vi "Parse Measured Data.vi"(6 "Waveform Template":waveform(dbl), 8 "error in":errorcluster, 9 "Current":dbl[](array[numeric]), 10 "Voltage":dbl[](array[numeric]), 11 "Electronic Load in":refnum<class "Electronic Load.lvclass">) -> (0 "error out":errorcluster, 3 "Electronic Load out":refnum<class "Electronic Load.lvclass">)   [LabVIEW 2019, in "Electronic Load.lvlib" / "Electronic Load.lvclass"]
uses:
  Library/Electronic Load.lvclass
  C:/Users/Public/Documents/Development/builds/Instruments/Instruments.lvlibp/Library/Instruments.lvclass
  Library/Electronic Load.lvclass/Electronic Load.ctl
  GUI/Read Measured_Table.vi
  GUI/Read Channel_Names.vi
  Accessors/Status/Read Status_Flags.vi
  GUI/Write Measured_Table.vi
  builds/Instruments/Instruments.lvlibp/Accessors/Write Measured.vi
  builds/Instruments/Instruments.lvlibp/Library/Instruments.lvclass
panel:
  in  "Waveform Labels":T1(ring)
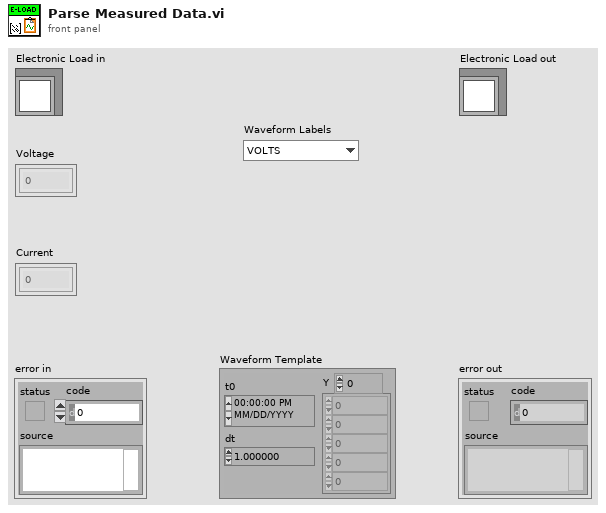
[diagram p1: front panel]
types:
  T1 = enum16{"VOLTS", "AMPS", "POWER", "OUTPUT", "OCP", "OVP"}
  T2 = typedef "Electronic Load.lvlib/Electronic Load.lvclass/Status_Flags.ctl" = cluster{"Interlock":bool, "OVP":bool, "OCP":bool, "Output":bool}
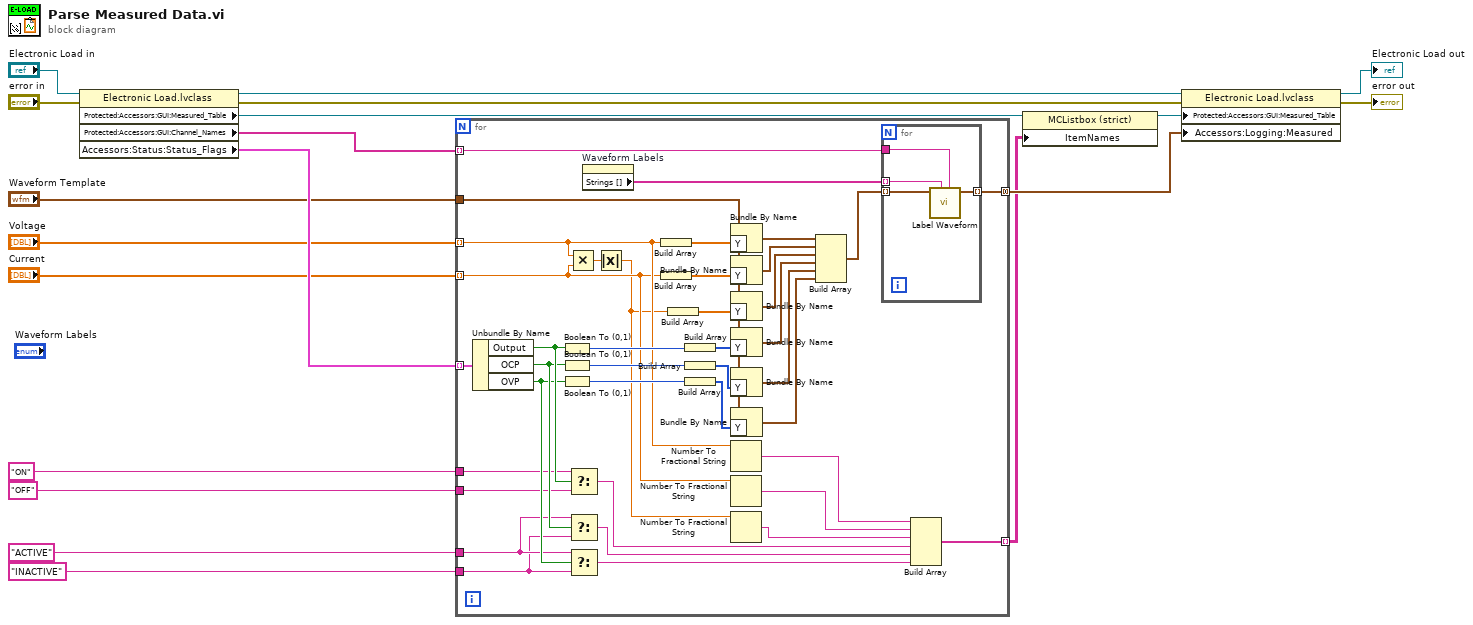
[diagram p0: block diagram]
diagram:
  n1 = property class="Electronic Load.lvclass"(reference="Electronic Load in", error in="error in") -> (reference out=w15:refnum<class "Electronic Load.lvclass">, error out=w14:errorcluster, "Protected:Accessors:GUI:Measured_Table"=w2:refnum<vi>, "Protected:Accessors:GUI:Channel_Names"=w9:string[], "Accessors:Status:Status_Flags"=w13:T2[])
  n2 = for {
    tunnel: w9 -> [w20] mode=indexing
    tunnel: w13 -> [w58] mode=indexing
    tunnel: "Waveform Template" -> [w30]
    tunnel: "Voltage" -> [w24] mode=indexing
    tunnel: "Current" -> [w23] mode=indexing
    tunnel: [w53] -> w8 mode=concatenating
    tunnel: "ACTIVE" -> [w46]
    tunnel: "INACTIVE" -> [w45]
    tunnel: "ON" -> [w44]
    tunnel: "OFF" -> [w43]
    tunnel: [w37] -> w1 mode=indexing
    n3 = Unbundle By Name(w58) -> ("Output"=w49:bool, "OCP"=w48:bool, "OVP"=w47:bool)
    n4 = Boolean To (0,1)(Boolean=w49) -> (0, 1=w57:i16)
    n5 = Boolean To (0,1)(Boolean=w48) -> (0, 1=w55:i16)
    n6 = Boolean To (0,1)(Boolean=w47) -> (0, 1=w56:i16)
    n7 = Multiply(x=w24, y=w23) -> (x*y=w25:dbl)
    n8 = Select(t=w44, s=w49, f=w43) -> (s? t:f=w40:string)
    n9 = Select(t=w46, s=w48, f=w45) -> (s? t:f=w41:string)
    n10 = Select(t=w46, s=w47, f=w45) -> (s? t:f=w42:string)
    n11 = property on="Waveform Labels" class="Enum (strict)"() -> ("Strings []"=w54:string[])  [unwired: 2 in, 2 out]
    n12 = Absolute Value(x=w25) -> (abs(x)=w22:dbl)
    n13 = Build Array(w24) -> (w29:dbl[])
    n14 = Build Array(w23) -> (w28:dbl[])
    n15 = Build Array(w22) -> (w21:dbl[])
    n16 = Build Array(w57) -> (w52:i16[])
    n17 = Build Array(w55) -> (w51:i16[])
    n18 = Build Array(w56) -> (w50:i16[])
    n19 = Bundle By Name(cluster=w30, "Y"=w29) -> (w36:waveform(dbl))
    n20 = Bundle By Name(cluster=w30, "Y"=w28) -> (w31:waveform(dbl))
    n21 = Bundle By Name(cluster=w30, "Y"=w21) -> (w27:waveform(dbl))
    n22 = Bundle By Name(cluster=w30, "Y"=w52) -> (w35:waveform(dbl))
    n23 = Bundle By Name(cluster=w30, "Y"=w51) -> (w34:waveform(dbl))
    n24 = Bundle By Name(cluster=w30, "Y"=w50) -> (w33:waveform(dbl))
    n25 = Number To Fractional String(number=w24) -> (F-format string=w38:string)  [unwired: 3 in]
    n26 = Number To Fractional String(number=w23) -> (F-format string=w39:string)  [unwired: 3 in]
    n27 = Number To Fractional String(number=w22) -> (F-format string=w26:string)  [unwired: 3 in]
    n28 = Build Array(w36, w31, w27, w35, w34, w33) -> (w32:waveform(dbl)[])
    n29 = for {
      tunnel: w54 -> [w62] mode=indexing
      tunnel: w20 -> [w61]
      tunnel: [w60] -> w53 mode=indexing
      tunnel: w32 -> [w59] mode=indexing
      n30 = call "Label Waveform.vi"("Unique Channel Name"=w61, "Measurement"=w62, "Input waveform"=w59) -> ("Labelled Waveform"=w60:waveform(dbl))  [unwired: 8 in]
    }
    n31 = Build Array(w38, w39, w26, w40, w41, w42) -> (w37:string[])
  }
  n32 = property class="MCListbox (strict)"(reference=w2, "ItemNames"=w1) -> (reference out=w3:refnum<vi>)  [unwired: 1 in, 1 out]
  n33 = property class="Electronic Load.lvclass"(reference=w15, error in=w14, "Protected:Accessors:GUI:Measured_Table"=w3, "Accessors:Logging:Measured"=w8) -> (reference out=→"Electronic Load out":refnum<class "Electronic Load.lvclass">, error out=→"error out":errorcluster)
